vi "hourly.vi"(8 "error in (no error)":errorcluster) -> (0 "error out":errorcluster)   [LabVIEW 2017]
uses:
  <vilib>/Math Plots/3D Math Plots/3D Pie/3D Pie XCtrl/3D Pie.xctl
  <vilib>/addons/database/Connection.llb/DB Tools Open Connec (Path).vi
  <vilib>/addons/database/Connection.llb/Conn Execute.vi
  <vilib>/addons/database/Recordset.llb/Rec Fetch Recordset Data (R).vi
  <vilib>/addons/database/Recordset.llb/Rec Destroy - Connection.vi
  <vilib>/Math Plots/3D Math Plots/3D Pie/3D Pie Datatype/Public/Plot Helper (Vector).vi
  <vilib>/addons/database/NI_Database_API.lvlib
  <vilib>/Math Plots/3D Math Plots/3D Pie/3D Pie Datatype/3D Pie Datatype.lvclass
panel:
  out "Station list":string[](array[string])
  out "Station size":i32
  in  "Tab Control":T1(tab)
  out "Table":string[][](table)
  out "Production":refnum<class "3D Plot Datatype.lvclass">[](xcontrol)
  out "Rejection":refnum<class "3D Plot Datatype.lvclass">[](xcontrol)
  out "Station Count":i32
  out "All Shifts":bool
  in  "Cancel Button - Archive":bool
  in  "Download 2":bool
  in  "Get Rport 2":bool
  in  "Shift":string(combo)
  in  "Station":string(combo)
  in  "Date":timestamp format="%<%Y-%m-%d>T"
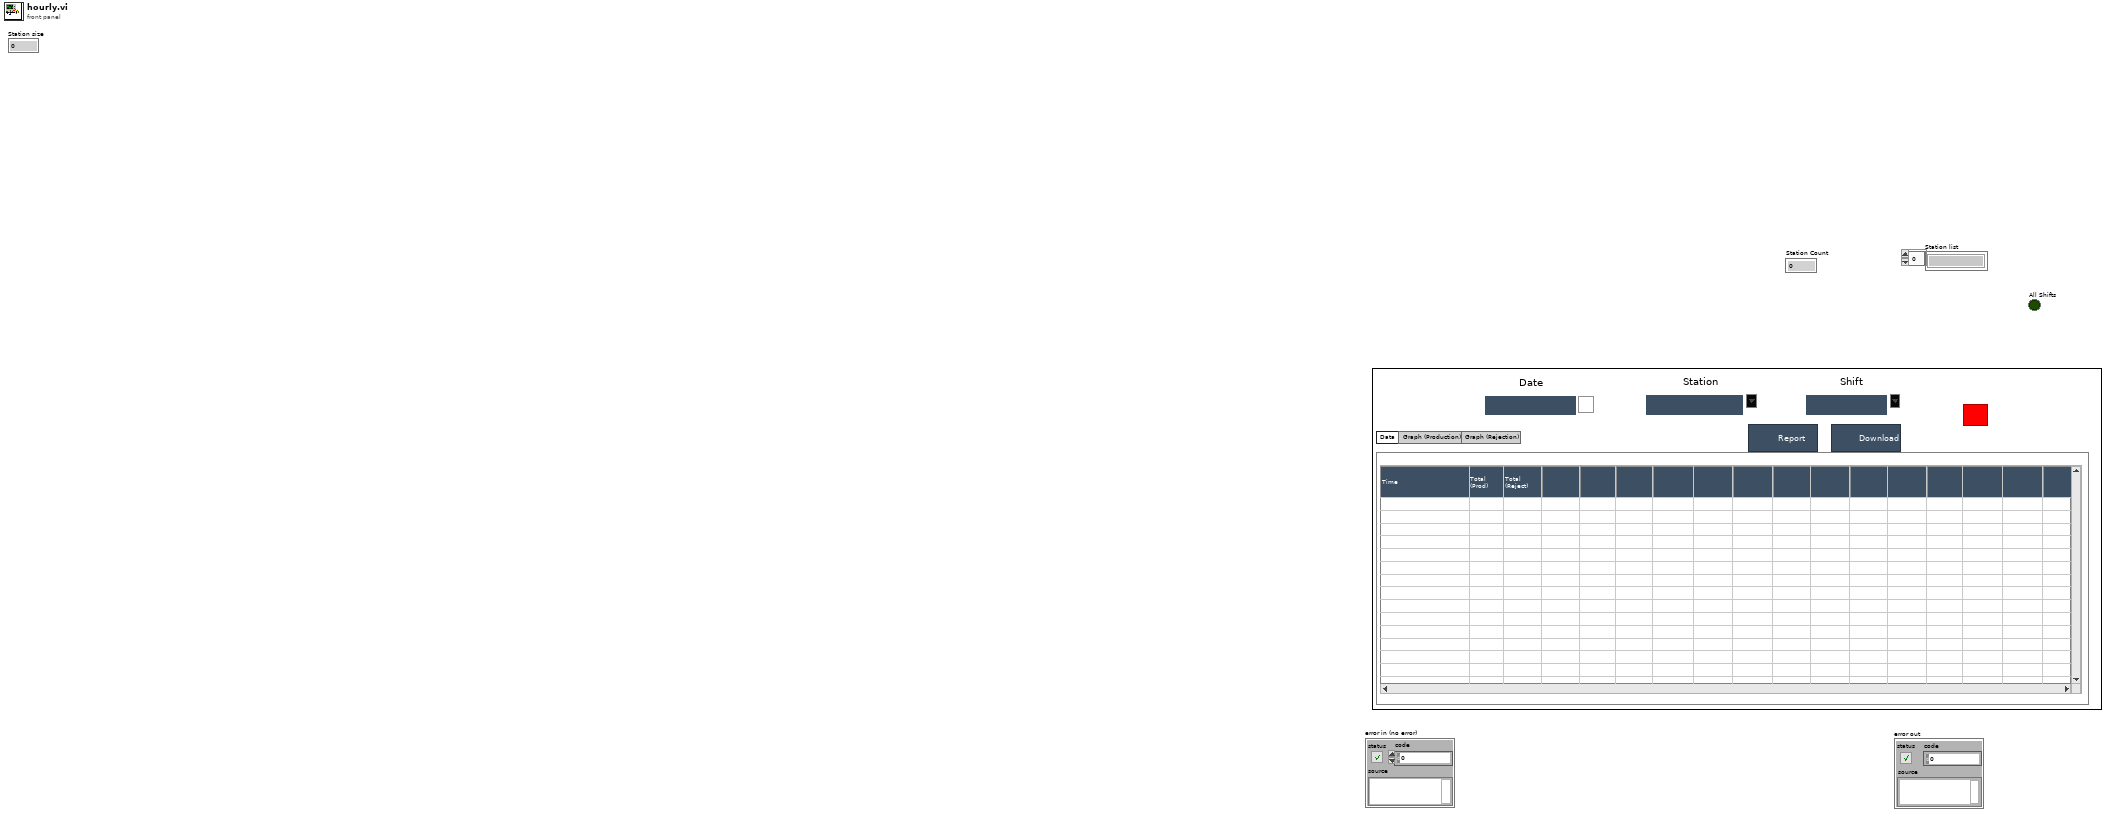
[diagram p1: front panel]
types:
  T1 = enum32{"Data", "Graph (Production)", "Graph (Rejection)"}
  T2 = typedef "NI_Database_API.lvlib/Conn ObjectReference.ctl" = refnum<k1>
  T3 = typedef "NI_Database_API.lvlib/Rec ObjectReference.ctl" = refnum<k1>
  T4 = typedef "LVDateTimeRec.ctl" = cluster{"fractional second":dbl, "second":i32, "minute":i32, "hour":i32, "day of month":i32, "month":i32, "year":i32, "day of week":i32, "day of year":i32, "DST":i32}
  T5 = enum32{"invalid app kind", "Development System", "Run Time System", "Student Edition", "Embedded LabVIEW", "Evaluation", "Custom"}
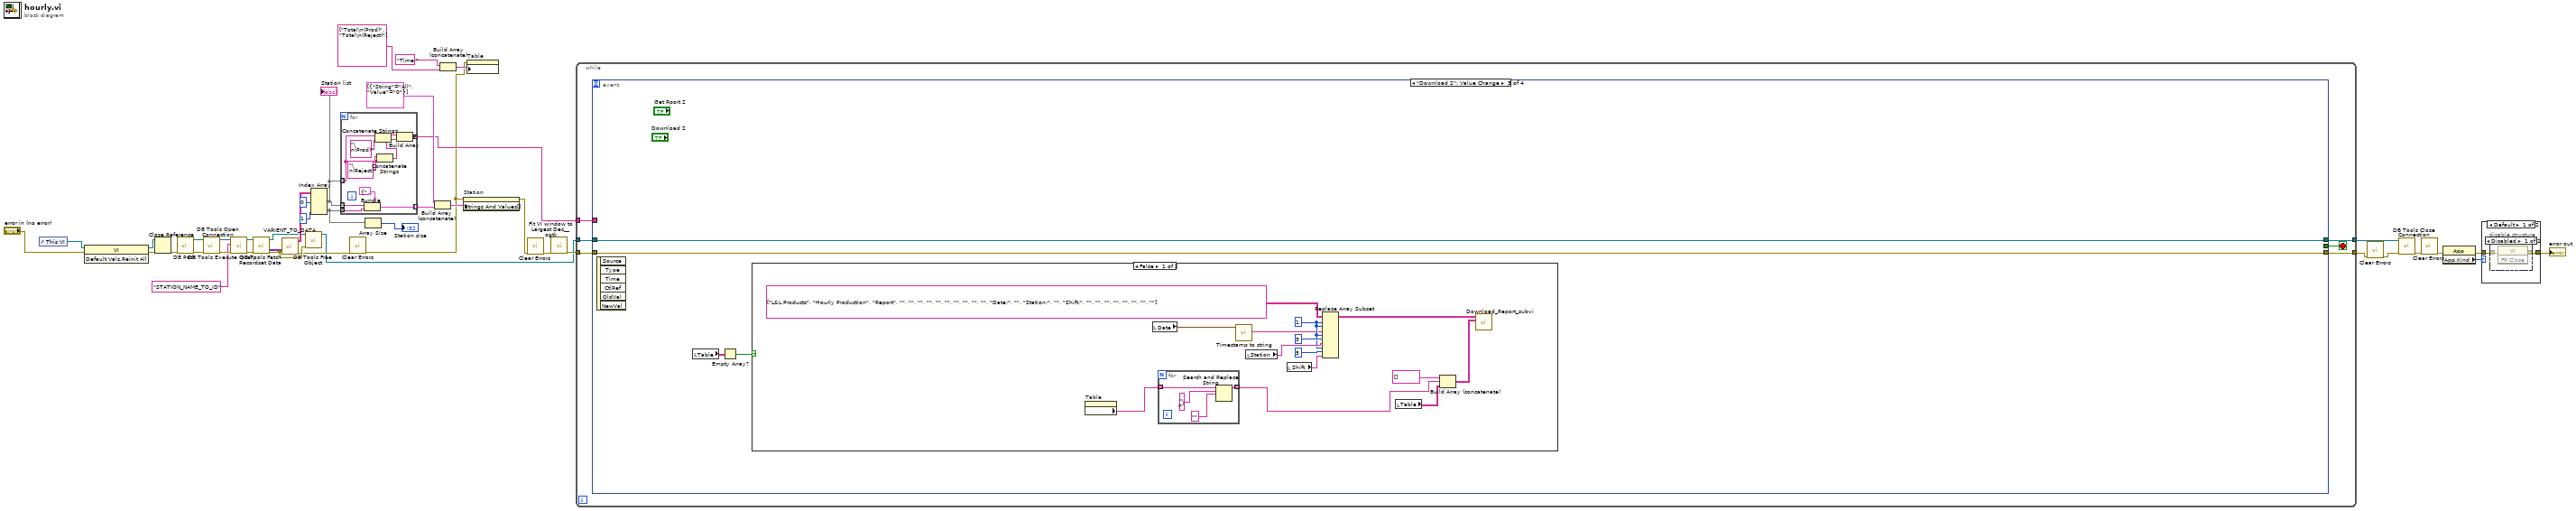
[diagram p0: block diagram]
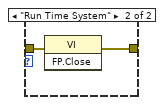
[diagram p3: hidden frame]
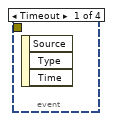
[diagram p4: hidden frame]
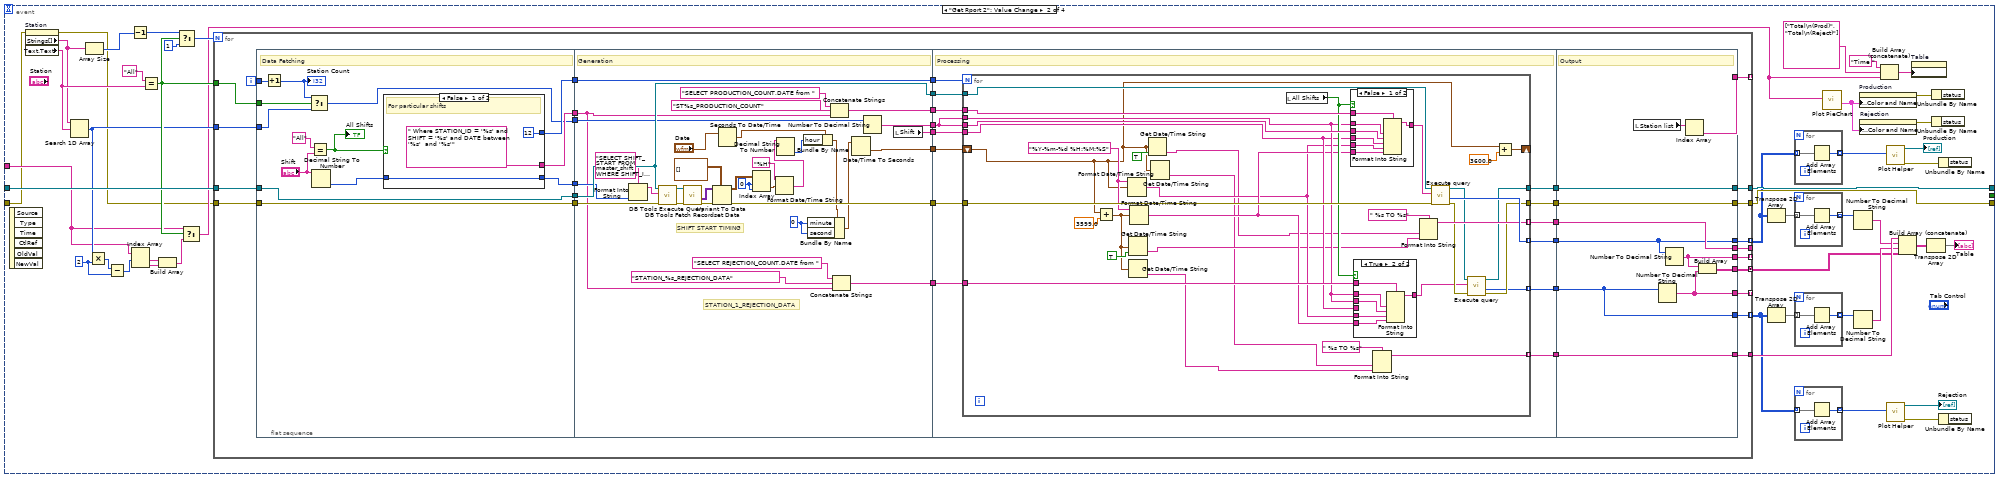
[diagram p5: hidden frame]
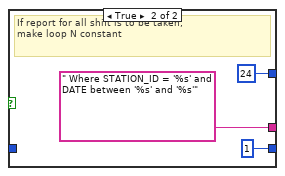
[diagram p6: hidden frame]
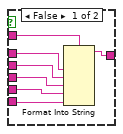
[diagram p7: hidden frame]
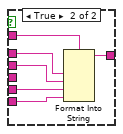
[diagram p8: hidden frame]
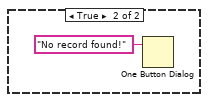
[diagram p9: hidden frame]
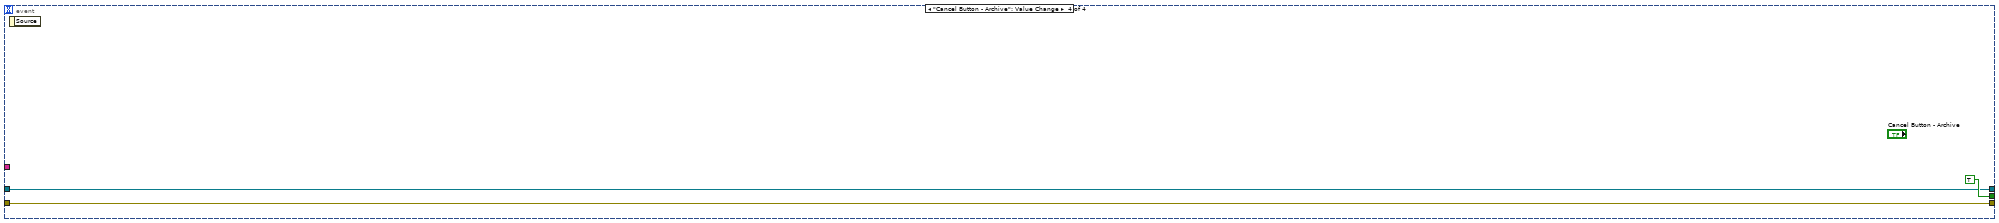
[diagram p10: hidden frame]
diagram:
  n1 = control-ref of="This VI"() -> (w36:refnum<vi>)
  n2 = invoke class="VI" method="Default Vals.Reinit All"(reference=w36, error in="error in (no error)") -> (reference out=w34:refnum<vi>, error out=w35:errorcluster)  [unwired: 1 in, 1 out]
  n3 = Close Reference(reference=w34, error in (no error)=w35) -> (error out=w33:errorcluster)
  n4 = call "DB Path.vi"("error in"=w33) -> ("error out"=w32:errorcluster, "DB Path"=w31:path)  [unwired: 9 in]
  n5 = call-poly <vilib>:"DB Tools Open Connection.vi"("error in (no error)"=w32, "connection information"=w31) -> ("error out"=w20:errorcluster, "connection reference"=w21:T2)  [unwired: 6 in]
  n6 = call-poly <vilib>:"DB Tools Execute Query.vi"("error in (no error)"=w20, "SQL query"="STATION_NAME_TO_ID", "connection reference"=w21) -> ("error out"=w29:errorcluster, "recordset reference"=w30:T3)  [unwired: 5 in]
  n7 = call-poly <vilib>:"DB Tools Fetch Recordset Data.vi"("error in (no error)"=w29, "recordset reference"=w30) -> ("error out"=w24:errorcluster, "recordset data"=w28:variant[][], "recordset reference out"=w22:T3)  [unwired: 3 in]
  n8 = call "VARIENT_TO_DATA.vi"("data"=w28, "error in (no error)"=w24) -> ("Table"=w25:string[][], "error out"=w23:errorcluster)  [unwired: 7 in]
  n9 = call-poly <vilib>:"DB Tools Free Object.vi"("error in (no error)"=w24, "recordset reference"=w22) -> ("connection reference"=w9:T2)  [unwired: 8 in, 1 out]
  n10 = Index Array(array=w25, index (col) #1=0 ("index (row)"), index (col) #2=1 ("index (col)")) -> (element #1=w8:string[], element #2=w15:string[])  [unwired: 2 in]
  "Station list" <- w8
  n11 = for {
    tunnel: w8 -> [w52] mode=indexing
    tunnel: w15 -> [w51] mode=indexing
    tunnel: [w49] -> w16 mode=indexing
    tunnel: w8 -> [w46] mode=indexing
    tunnel: [w43] -> w7 mode=concatenating
    n12 = Bundle(cluster=cluster{"String":string, "Value":string} {"String"="", "Value"=""}, "String"=w52, "Value"=w51) -> (w49:cluster{"String":string, "Value":string})
    n13 = Concatenate Strings(w46, "\n(Prod)" ("string")) -> (w44:string)
    n14 = Concatenate Strings(w46, "\n(Reject)" ("string")) -> (w45:string)
    n15 = Build Array(w44, w45) -> (w43:string[])
  }
  n16 = call <vilib>:"Clear Errors.vi"("error in (no error)"=w23) -> ("error out"=w1:errorcluster)  [unwired: 5 in, 1 out]
  n17 = Array Size(array=w15) -> (size(s)=→"Station size":i32)
  n18 = Build Array (concatenate)(cluster{"String":string, "Value":string}[] [{"String"="All", "Value"="0"}] ("array"), w16) -> (w18:cluster{"String":string, "Value":string}[])
  n19 = Build Array (concatenate)("Time ", string[] ["Total\n(Prod)", "Total\n(Reject)"]) -> (w2:string[])
  n20 = property on="Station" class="CmbBox"(error in=w1, "Strings And Values[]"=w18) -> (error out=w12:errorcluster)  [unwired: 1 in, 1 out]
  n21 = property on="Table" class="Tbl (strict)"(error in=w1, "Column Headers[]"=w2) -> ()  [unwired: 1 in, 2 out]
  n22 = call <vilib>:"Clear Errors.vi"("error in (no error)"=w12) -> ("error out"=w13:errorcluster)  [unwired: 5 in, 1 out]
  n23 = call <userlib>:"Fit VI window to Largest Dec__ogtk.vi"("error in (no error)"=w13) -> ("error out"=w10:errorcluster)  [unwired: 5 in, 1 out]
  n24 = while {
    tunnel: w10 -> [w55]
    tunnel: w9 -> [w54]
    tunnel: [w57] -> w5
    tunnel: [w56] -> w38
    tunnel: w7 -> [w53]
    stop <- w58 stop-if-true
    n25 = event shown="[2] \"Download 2\": Value Change" {
      selector: _ -> [_ _ _ _]
      dyn-events: _ -> [_ _ _ _]
      timeout: _ -> [_ _ _ _]
      tunnel: w54 -> [_ w104 w290 w311]
      tunnel: [_ _ _ TRUE] -> w58
      tunnel: [_ w102 w289 w310] -> w57
      tunnel: [_ w103 w290 w311] -> w56
      tunnel: w55 -> [_ w60 w289 w310]
      tunnel: w53 -> [_ w85 _ _]
      event Timeout {
        n26 = event-data() -> ()  [unwired: 1 in, 3 out]
      }
      event "Get Rport 2": Value Change {
        w88 = 2 ("y")
        n27 = event-data() -> ()  [unwired: 1 in, 6 out]
        n28 = property on="Station" class="CmbBox"(error in=w60) -> (error out=w61:errorcluster, "Strings[]"=w59:string[], "Text.Text"=w62:string)  [unwired: 1 in, 1 out]
        n29 = Search 1D Array(1D array=w59, element=w62) -> (index of element=w92:i32)  [unwired: 1 in]
        n30 = Array Size(array=w59) -> (size(s)=w98:i32)
        n31 = Multiply(x=w92, y=w88) -> (x*y=w87:i32)
        n32 = Subtract(x=w87, y=w88) -> (x-y=w86:i32)
        n33 = Decrement(x=w98) -> (x-1=w97:i32)
        n34 = Index Array(array=w85, index #1=w86) -> (element #1=w90:string, element #2=w91:string)  [unwired: 1 in]
        n35 = Equal?(x="All", y=w62) -> (x = y?=w93:bool)
        n36 = Build Array(w90, w91) -> (w89:string[])
        n37 = Select(t=w97, s=w93, f=1) -> (s? t:f=w100:i32)
        n38 = Select(t=w85, s=w93, f=w89) -> (s? t:f=w83:string[])
        n39 = for {
          N: w100 -> [_]
          tunnel: w93 -> [w127]
          tunnel: w92 -> [w126]
          tunnel: [w123] -> _
          tunnel: [w124] -> _ mode=indexing
          tunnel: [w122] -> _ mode=indexing
          tunnel: [w121] -> w66 mode=indexing
          tunnel: [w118] -> _ mode=indexing
          tunnel: [w117] -> w70 mode=concatenating
          tunnel: [w116] -> w78
          tunnel: [w114] -> w65 mode=indexing
          tunnel: w61 -> [w128]
          tunnel: [w129] -> w102
          tunnel: w104 -> [w131]
          tunnel: [w130] -> w103
          i -> [w125]
          n40 = flat-sequence {
            tunnel: w128 -> [w161]
            tunnel: w131 -> [w156]
            tunnel: [w159] -> w147
            tunnel: [w160] -> w146
            tunnel: [w161] -> w145
            tunnel: [w156] -> w144
            tunnel: [w152] -> w143
            tunnel: [w158] -> w142
            tunnel: w127 -> [w149]
            tunnel: w126 -> [w155]
            tunnel: w125 -> [w154]
            tunnel: [w195] -> w141
            tunnel: [w201] -> w140
            tunnel: [w200] -> w139
            tunnel: [w199] -> w138
            tunnel: [w192] -> w137
            tunnel: [w198] -> w136
            tunnel: w142 -> [w180]
            tunnel: w143 -> [w181]
            tunnel: w144 -> [w199]
            tunnel: w145 -> [w184]
            tunnel: w146 -> [w177]
            tunnel: w147 -> [w198]
            tunnel: [w176] -> w120
            tunnel: [w171] -> w113
            tunnel: [w214] -> w135
            tunnel: [w213] -> w134
            tunnel: [w211] -> w133
            tunnel: [w210] -> w132
            tunnel: w141 -> [w215]
            tunnel: w140 -> [w212]
            tunnel: w139 -> [w207]
            tunnel: w138 -> [w209]
            tunnel: w137 -> [w208]
            tunnel: w136 -> [w204]
            tunnel: w120 -> [w206]
            tunnel: [w205] -> w119
            tunnel: [w203] -> w115
            tunnel: w113 -> [w202]
            tunnel: [w286] -> w130
            tunnel: w135 -> [w285]
            tunnel: w134 -> [w286]
            tunnel: w133 -> [w278]
            tunnel: w132 -> [w283]
            tunnel: [w285] -> w129
            tunnel: [w282] -> w124
            tunnel: [w283] -> w123
            tunnel: [w284] -> w122
            tunnel: [w278] -> w121
            tunnel: w119 -> [w277]
            tunnel: [w281] -> w118
            tunnel: [w280] -> w117
            tunnel: [w279] -> w116
            tunnel: w115 -> [w279]
            tunnel: [w277] -> w114
            frame #0 {
              # "Data Fetching"
              n41 = Increment(x=w154) -> (x+1=w153:i32)
              "Station Count" <- w153
              n42 = Select(t=w153, s=w149, f=w155) -> (s? t:f=w152:i32)
              n43 = Equal?(x="All", y="Shift") -> (x = y?=w148:bool)
              "All Shifts" <- w148
              n44 = Decimal String To Number(string="Shift") -> (number=w157:i32)  [unwired: 2 in, 1 out]
              n45 = case shown="False" w148 {
                tunnel: [" Where STATION_ID = '%s' and SHIFT = '%s' and DATE between '%s'  and '%s'" ("format string") " Where STATION_ID = '%s' and DATE between '%s' and '%s'" ("format string")] -> w160
                tunnel: [12 ("Shift Hrs") 24 ("Shift Hrs")] -> w159
                tunnel: [w163 1] -> w158
                tunnel: w157 -> [w163 _]
                frame False {
                  # "For particular shifts"
                }
                frame True {
                  # "If report for all shift is to be taken,\nmake loop N constant"
                }
              }
            }
            frame #1 {
              w168 = 0
              w188 = 0 ("index (row)")
              # "SHIFT START TIMING"
              # "STATION_1_REJECTION_DATA"
              # "Generation"
              n46 = Format Into String(format string="SELECT SHIFT_START FROM master_shift WHERE SHIFT_ID = %d  " ("SQL query"), w180) -> (resulting string=w186:string)  [unwired: 2 in, 1 out]
              n47 = call-poly <vilib>:"DB Tools Execute Query.vi"("error in (no error)"=w184, "SQL query"=w186, "connection reference"=w199) -> ("error out"=w183:errorcluster, "recordset reference"=w182:T3)  [unwired: 5 in]
              n48 = call-poly <vilib>:"DB Tools Fetch Recordset Data.vi"("error in (no error)"=w183, "recordset reference"=w182) -> ("error out"=w191:errorcluster, "recordset data"=w189:variant[][])  [unwired: 3 in, 1 out]
              n49 = Variant To Data(error in=w191, type=timestamp[][] [] ("From Date 2"), Variant=w189) -> (data=w190:timestamp[][], error out=w201:errorcluster)
              n50 = Seconds To Date/Time(time stamp (now)="Date") -> (date time rec=w175:T4)  [unwired: 1 in]
              n51 = Index Array(array=w190, index (row)=w188, index (col)=w188) -> (element=w194:timestamp)
              n52 = Format Date/Time String(time format string (%c)="%H", seconds (now)=w194) -> (date/time string=w174:string)  [unwired: 1 in]
              n53 = Decimal String To Number(string=w174) -> (number=w173:i32)  [unwired: 2 in, 1 out]
              n54 = Bundle By Name(cluster=w175, "hour"=w173) -> (w170:T4)
              n55 = Bundle By Name(cluster=w170, "minute"=w168, "second"=w168) -> (w169:T4)
              n56 = Concatenate Strings("SELECT PRODUCTION_COUNT,DATE from " ("format string"), "ST%s_PRODUCTION_COUNT", w177) -> (w195:string)
              n57 = Concatenate Strings("SELECT REJECTION_COUNT,DATE from " ("format string"), "STATION_%s_REJECTION_DATA", w177) -> (w176:string)
              n58 = Date/Time To Seconds(2:w169) -> (0:w171:timestamp)  [unwired: 1 in]
              n59 = Number To Decimal String(number=w181) -> (decimal integer string=w200:string)  [unwired: 1 in]
              n60 = local read "Shift"() -> (w192:string)
            }
            frame #2 {
              # "Processing"
              n61 = for {
                N: w204 -> [_]
                tunnel: w215 -> [w249]
                tunnel: w209 -> [w244]
                tunnel: w208 -> [w235]
                tunnel: w207 -> [w243]
                tunnel: [w247] -> w211 mode=indexing
                tunnel: [w245] -> w210 mode=indexing
                tunnel: [w239] -> w213
                tunnel: w207 -> [w236]
                tunnel: w206 -> [w237]
                tunnel: [w234] -> w205 mode=indexing
                tunnel: [w230] -> w203 mode=indexing
                tunnel: w212 -> [w248]
                tunnel: [w240] -> w214
                shift-right: [w228] -> _
                shift-left: w202 -> [w218]
                w227 = "%Y-%m-%d %H:%M:%S" ("time format string (%c)")
                n62 = Add(x=w218, y=3599.0 ("x-y")) -> (x+y=w221:timestamp)
                n63 = Format Date/Time String(time format string (%c)=w227, seconds (now)=w218) -> (date/time string=w222:string)  [unwired: 1 in]
                n64 = Get Date/Time String(seconds (now)=w221, want seconds? (F)=TRUE) -> (time string=w220:string)  [unwired: 1 in, 1 out]
                n65 = Get Date/Time String(seconds (now)=w221) -> (time string=w219:string)  [unwired: 2 in, 1 out]
                n66 = Format Date/Time String(time format string (%c)=w227, seconds (now)=w221) -> (date/time string=w225:string)  [unwired: 1 in]
                n67 = Get Date/Time String(seconds (now)=w218, want seconds? (F)=TRUE) -> (time string=w217:string)  [unwired: 1 in, 1 out]
                n68 = Get Date/Time String(seconds (now)=w218) -> (time string=w216:string)  [unwired: 2 in, 1 out]
                n69 = local read "All Shifts"() -> (w238:bool)
                n70 = case shown="False" w238 {
                  tunnel: w249 -> [w269 w275]
                  tunnel: [w268 w274] -> w233
                  tunnel: w235 -> [w267 _]
                  tunnel: w222 -> [w266 w273]
                  tunnel: w225 -> [w265 w272]
                  tunnel: w243 -> [w264 w271]
                  tunnel: w236 -> [w263 w270]
                  frame False {
                    n71 = Format Into String(format string=w269, w263, w264, w267, w266, w265) -> (resulting string=w268:string)  [unwired: 2 in, 1 out]
                  }
                  frame True {
                    n72 = Format Into String(format string=w275, w270, w271, w273, w272) -> (resulting string=w274:string)  [unwired: 2 in, 1 out]
                  }
                }
                n73 = case shown="True" w238 {
                  tunnel: w237 -> [w256 w262]
                  tunnel: [w255 w261] -> w232
                  tunnel: w235 -> [w254 _]
                  tunnel: w222 -> [w253 w260]
                  tunnel: w225 -> [w252 w259]
                  tunnel: w236 -> [w251 w258]
                  tunnel: w236 -> [w250 w257]
                  frame False {
                    n74 = Format Into String(format string=w256, w250, w251, w254, w253, w252) -> (resulting string=w255:string)  [unwired: 2 in, 1 out]
                  }
                  frame True {
                    n75 = Format Into String(format string=w262, w257, w258, w260, w259) -> (resulting string=w261:string)  [unwired: 2 in, 1 out]
                  }
                }
                n76 = Format Into String(format string=" %s TO %s", w216, w219) -> (resulting string=w230:string)  [unwired: 2 in, 1 out]
                n77 = Format Into String(format string=" %s TO %s", w217, w220) -> (resulting string=w245:string)  [unwired: 2 in, 1 out]
                n78 = call "Execute query.vi"("error in (no error)"=w248, "String"=w233, "connection reference"=w244) -> ("error out"=w241:errorcluster, "Production Count"=w247:i32, "connection reference 2"=w242:T2)  [unwired: 3 in, 3 out]
                n79 = call "Execute query.vi"("error in (no error)"=w241, "String"=w232, "connection reference"=w242) -> ("error out"=w240:errorcluster, "Production Count"=w234:i32, "connection reference 2"=w239:T2)  [unwired: 3 in, 3 out]
                n80 = Add(x=w218, y=3600.0 ("x-y")) -> (x+y=w228:timestamp)
              }
            }
            frame #3 {
              # "Output"
              n81 = local read "Station list"() -> (w276:string[])
              n82 = Number To Decimal String(number=w277) -> (decimal integer string=w281:string[])  [unwired: 1 in]
              n83 = Number To Decimal String(number=w278) -> (decimal integer string=w282:string[])  [unwired: 1 in]
              n84 = Index Array(array=w276) -> (element=w284:string)  [unwired: 1 in]
              n85 = Build Array(w282, w281) -> (w280:string[][])
            }
          }
        }
        n86 = Transpose 2D Array(2D array=w66) -> (transposed array=w74:i32[][])
        n87 = Transpose 2D Array(2D array=w65) -> (transposed array=w73:i32[][])
        n88 = for {
          tunnel: w66 -> [w112] mode=indexing
          tunnel: [w111] -> w77 mode=indexing
          n89 = Add Array Elements(numeric array=w112) -> (sum=w111:i32)
        }
        n90 = for {
          tunnel: w74 -> [w110] mode=indexing
          tunnel: [w109] -> w75 mode=indexing
          n91 = Add Array Elements(numeric array=w110) -> (sum=w109:i32)
        }
        n92 = for {
          tunnel: w73 -> [w108] mode=indexing
          tunnel: [w107] -> w72 mode=indexing
          n93 = Add Array Elements(numeric array=w108) -> (sum=w107:i32)
        }
        n94 = for {
          tunnel: w65 -> [w106] mode=indexing
          tunnel: [w105] -> w69 mode=indexing
          n95 = Add Array Elements(numeric array=w106) -> (sum=w105:i32)
        }
        n96 = call "Plot PieChart.vi"("Label"=w83) -> ("Labelling"=w63:cluster{dbl, "String":string}[])  [unwired: 10 in]
        n97 = Number To Decimal String(number=w75) -> (decimal integer string=w76:string[])  [unwired: 1 in]
        n98 = Number To Decimal String(number=w72) -> (decimal integer string=w71:string[])  [unwired: 1 in]
        n99 = property on="Production" class="3D Pie (strict)"("Plot Specific:Color and Name"=w63) -> (error out=w81:errorcluster)  [unwired: 2 in, 1 out]
        n100 = property on="Rejection" class="3D Pie (strict)"("Plot Specific:Color and Name"=w63) -> (error out=w64:errorcluster)  [unwired: 2 in, 1 out]
        n101 = Build Array (concatenate)("Time ", string[] ["Total\n(Prod)", "Total\n(Reject)"], w83) -> (w94:string[])
        n102 = call-poly <vilib>:"Plot Helper.vi"("x vector"=w77) -> ("error out"=w84:errorcluster, "3D Plot lvclass Array out"=→"Production":refnum<class "3D Plot Datatype.lvclass">[])  [unwired: 2 in, 7 out]
        n103 = call-poly <vilib>:"Plot Helper.vi"("x vector"=w69) -> ("error out"=w68:errorcluster, "3D Plot lvclass Array out"=→"Rejection":refnum<class "3D Plot Datatype.lvclass">[])  [unwired: 2 in, 7 out]
        n104 = Build Array (concatenate)(w78, w76, w71, w70) -> (w95:string[][])
        n105 = property on="Table" class="Tbl (strict)"("Column Headers[]"=w94) -> ()  [unwired: 2 in, 2 out]
        n106 = Transpose 2D Array(2D array=w95) -> (transposed array=→"Table":string[][])
        n107 = Unbundle By Name(w81) -> ()  [unwired: 1 out]
        n108 = Unbundle By Name(w64) -> ()  [unwired: 1 out]
        n109 = Unbundle By Name(w84) -> ()  [unwired: 1 out]
        n110 = Unbundle By Name(w68) -> ()  [unwired: 1 out]
      }
      event "Download 2": Value Change {
        n111 = event-data() -> ()  [unwired: 1 in, 6 out]
        n112 = local read "Table"() -> (w288:string[][])
        n113 = Empty Array?(array=w288) -> (empty?=w287:bool)
        n114 = case shown="False" w287 {
          frame False {
            w300 = 1 ("index (row)")
            n115 = property on="Table" class="Tbl (strict)"() -> ("Column Headers[]"=w292:string[])  [unwired: 2 in, 2 out]
            n116 = local read "Date"() -> (w297:timestamp)
            n117 = for {
              tunnel: w292 -> [w308] mode=indexing
              tunnel: [w305] -> w291 mode=indexing
              n118 = Search and Replace String(input string=w308, search string="\n", replace string="" ("replace string (\"\")")) -> (result string=w305:string)  [unwired: 5 in, 3 out]
            }
            n119 = call "Timestamp to string.vi"("time stamp"=w297) -> ("Date"=w296:string)  [unwired: 8 in, 2 out]
            n120 = local read "Station"() -> (w301:string)
            n121 = local read "Shift"() -> (w298:string)
            n122 = Replace Array Subset(array=string[][] [["L&L Products", "Hourly Production", "Report", "", "", "", "", "", "", "", "", "", ""], ["Date:", "", "Station:", "", "Shift:", "", "", "", "", "", "", "", ""]] ("Column Header Strings[]"), new element #1=w296, index (row) #1=w300, index (col) #1=w300, new element #2=w301, index (row) #2=w300, index (col) #2=3 ("disabled index (col)"), new element #3=w298, index (row) #3=w300, index (col) #3=5 ("disabled index (col)")) -> (w303:string[][])
            n123 = local read "Table"() -> (w294:string[][])
            n124 = Build Array (concatenate)(string[] [] ("element"), w291, w294) -> (w293:string[][])
            n125 = call "Download_Report_subvi.vi"("Value"=w293, "Column Header Strings[]"=w303) -> ()  [unwired: 9 in, 1 out]
          }
          frame True {
            n126 = One Button Dialog(message="No record found!") -> ()  [unwired: 1 in, 1 out]
          }
        }
      }
      event "Cancel Button - Archive": Value Change {
        n127 = event-data() -> ()  [unwired: 1 in, 1 out]
      }
    }
  }
  n128 = call <vilib>:"Clear Errors.vi"("error in (no error)"=w5) -> ("error out"=w6:errorcluster)  [unwired: 5 in, 1 out]
  n129 = call <vilib>:"DB Tools Close Connection.vi"("error in (no error)"=w6, "connection reference"=w38) -> ("error out"=w40:errorcluster)  [unwired: 5 in]
  n130 = call <vilib>:"Clear Errors.vi"("error in (no error)"=w40) -> ("error out"=w39:errorcluster)  [unwired: 5 in, 1 out]
  n131 = property class="App"(error in=w39) -> (error out=w41:errorcluster, "App.Kind"=w42:T5)  [unwired: 1 in, 1 out]
  n132 = case shown="Default" w42 {
    tunnel: w41 -> [w314 w318]
    tunnel: [w313 w317] -> w37
    frame Default {
      n133 = disable-structure shown="Disabled" {
        disable-tunnel: w314 -> [w316 _]
        disable-tunnel: [w315 _] -> w313
        frame Disabled {
          n134 = invoke class="VI" method="FP.Close"(error in=w316) -> (error out=w315:errorcluster)  [unwired: 2 in, 2 out]
        }
        frame Enabled {
        }
      }
    }
    frame "Run Time System" {
      n135 = invoke class="VI" method="FP.Close"(error in=w318) -> (error out=w317:errorcluster)  [unwired: 2 in, 2 out]
    }
  }
  "error out" <- w37
